vi "Save_In_2D_Array.vi"(1 "Vert":dbl[](array[numeric]), 2 "Horz":dbl[](array[numeric])) -> (0 "Array":dbl[][](array[numeric]))   [LabVIEW 2019]
doc: "Convert two separate 1D arrays to a single 2D array\n\nR. Sheehan 21 - 2 - 2017"
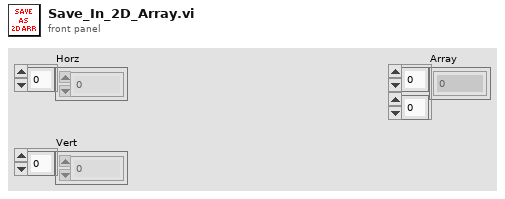
[diagram p1: front panel]
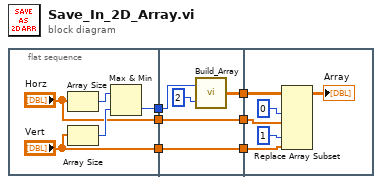
[diagram p0: block diagram]
diagram:
  n1 = flat-sequence {
    tunnel: [w9] -> w6
    tunnel: ["Vert"] -> w3
    tunnel: ["Horz"] -> w1
    tunnel: w6 -> [w12]
    tunnel: [w16] -> w5
    tunnel: [w15] -> w4
    tunnel: w3 -> [w15]
    tunnel: [w14] -> w2
    tunnel: w1 -> [w14]
    tunnel: w5 -> [w22]
    tunnel: w4 -> [w20]
    tunnel: w2 -> [w21]
    frame #0 {
      n2 = Array Size(array="Horz") -> (size(s)=w11:i32)
      n3 = Array Size(array="Vert") -> (size(s)=w10:i32)
      n4 = Max & Min(x=w11, y=w10) -> (min(x,y)=w9:i32)  [unwired: 1 out]
    }
    frame #1 {
      n5 = call "Build_Array.vi"("Ncolumns"=2 ("Nrows"), "Nrows"=w12) -> ("Array"=w16:dbl[][])
    }
    frame #2 {
      n6 = Replace Array Subset(array=w22, new element #1=w21, index (col) #1=0 ("index (row)"), new element #2=w20, index (col) #2=1 ("index (row)")) -> (→"Array":dbl[][])  [unwired: 2 in]
    }
  }
